vi "Create Map from Values Indexes to Channel and Label Indexes.vi"(8 "error in":errorcluster, 11 "RT hardware channels":T2[](array[typedef]) {"labels settings for RT"."Label Timestamp Channel Data Reference" format="%.0x"; "labels settings for RT"."Word Initial Raw Value" format="%032.0f"; "labels settings for RT"."Label Disable/Trigger Channel Reference" format="%.0x"; "labels settings for RT"."parameter driver data"."Tx parameter refs" format="%.0x"; "labels settings for RT"."parameter driver data"."Rx block data refs"."Data Reference" format="%.0x"; "labels settings for RT"."SDI" format="%02b"; "labels settings for RT"."label" format="%.0o"}) -> (0 "error out":errorcluster, 3 "map":T1)   [LabVIEW 2020, in "Ballard ARINC 429 Engine.lvlib" / "Custom Device.lvlib"]
uses:
  Custom Device.lvlib
  Shared/RT Hardware Channel Settings.ctl
  Shared/RT Label Settings.ctl
  Shared/Label.ctl
  Shared/RT Parameters.ctl
  Shared/Parameter Definition.ctl
  Encoding and Decoding/Encoding.ctl
  <vilib>/NI VeriStand/Custom Device API/Block Data Reference.ctl
  <vilib>/NI VeriStand/Custom Device API/Data Reference.ctl
  <vilib>/NI VeriStand/Custom Device API/Custom Device Item Ref.ctl
  Shared/Transfer Type.ctl
  Shared/Map of Values Indexes to Channel and Label Indexes.ctl
  Encoding and Decoding/Encoding and Decoding.lvlib
  <vilib>/NI VeriStand/Custom Device API/Custom Device API.lvlib
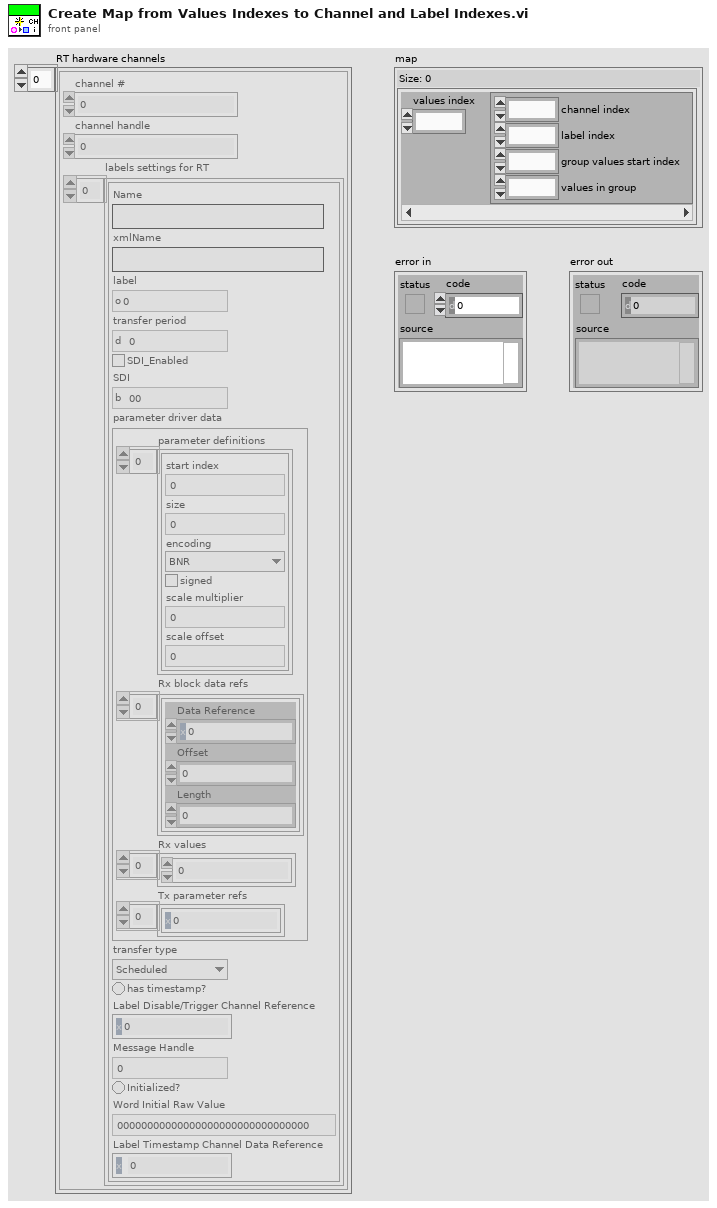
[diagram p1: front panel]
types:
  T1 = typedef "Map of Values Indexes to Channel and Label Indexes.ctl" = map{i32, cluster{"channel index":i32, "label index":i32, "group values start index":i32, "values in group":i32}}
  T2 = typedef "RT Hardware Channel Settings.ctl" = cluster{"channel #":u16, "channel handle":u64, "labels settings for RT":T3[]}
  T3 = typedef "RT Label Settings.ctl" = cluster{"Name":string, "xmlName":string, "label":T4, "transfer period":u32, "SDI_Enabled":bool, "SDI":u8, "parameter driver data":T5, "transfer type":T11, "has timestamp?":bool, "Label Disable/Trigger Channel Reference":T10, "Message Handle":u64, "Initialized?":bool, "Word Initial Raw Value":u32, "Label Timestamp Channel Data Reference":T9}
  T4 = typedef "Label.ctl" = u8
  T5 = typedef "RT Parameters.ctl" = cluster{"parameter definitions":T6[], "Rx block data refs":T8[], "Rx values":dbl[], "Tx parameter refs":T10[]}
  T6 = typedef "Parameter Definition.ctl" = cluster{"start index":i32, "size":i32, "encoding":T7, "signed":bool, "scale multiplier":dbl, "scale offset":dbl}
  T7 = typedef "Encoding and Decoding.lvlib/Encoding.ctl" = enum16{"BNR", "BCD", "Discrete"}
  T8 = typedef "Custom Device API.lvlib/Block Data Reference.ctl" = cluster{"Data Reference":T9, "Offset":u64, "Length":u64}
  T9 = typedef "Custom Device API.lvlib/Data Reference.ctl" = i32
  T10 = typedef "Custom Device API.lvlib/Custom Device Item Ref.ctl" = u64
  T11 = typedef "Transfer Type.ctl" = enum16{"Scheduled", "Acyclic", "Block", "Strobe"}
  T12 = cluster{"channel index":i32, "label index":i32, "group values start index":i32, "values in group":i32}
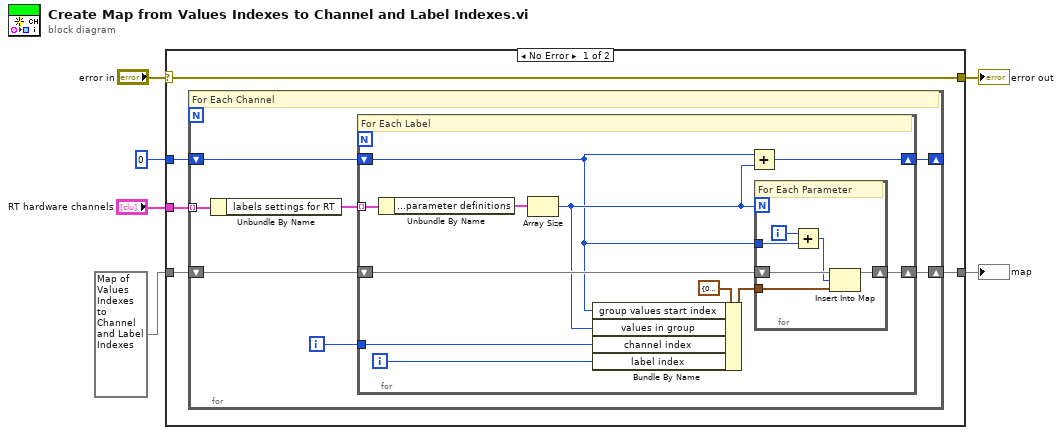
[diagram p0: block diagram]
diagram:
  n1 = case shown="No Error" "error in" {
    selector: "error in" -> [w7 w37]
    tunnel: "RT hardware channels" -> [w11 _]
    tunnel: 0 -> [w10 _]
    tunnel: T1 {} ("map") -> [w9 w36]
    tunnel: [w8 w36] -> w3
    tunnel: [w7 w37] -> w1
    frame No Error {
      n2 = for {
        tunnel: w11 -> [w18] mode=indexing
        shift-right: [w12] -> _
        shift-left: w10 -> [w14]
        shift-right: [w15] -> w8
        shift-left: w9 -> [w16]
        i -> [w13]
        # "For Each Channel"
        n3 = Unbundle By Name(w18) -> ("labels settings for RT"=w17:T3[])
        n4 = for {
          tunnel: w17 -> [w29] mode=indexing
          shift-right: [w26] -> w15
          shift-left: w16 -> [w27]
          tunnel: w13 -> [w25]
          shift-right: [w20] -> w12
          shift-left: w14 -> [w19]
          i -> [w24]
          # "For Each Label"
          n5 = Unbundle By Name(w29) -> ("parameter driver data.parameter definitions"=w28:T6[])
          n6 = Array Size(array=w28) -> (size(s)=w22:i32)
          n7 = Bundle By Name(cluster=T12 {"channel index"=0, "label index"=0, "group values start index"=0, "values in group"=0} ("value"), "group values start index"=w19, "values in group"=w22, "channel index"=w25, "label index"=w24) -> (w21:T12)
          n8 = Add(x=w19, y=w22) -> (x+y=w20:i32)
          n9 = for {
            N: w22 -> [_]
            shift-right: [w34] -> w26
            shift-left: w27 -> [w35]
            tunnel: w19 -> [w32]
            tunnel: w21 -> [w31]
            i -> [w33]
            # "For Each Parameter"
            n10 = Add(x=w33, y=w32) -> (x+y=w30:i32)
            n11 = Insert Into Map(map in=w35, key=w30, value=w31) -> (map out=w34:T1)  [unwired: 2 out]
          }
        }
      }
    }
    frame Error {
    }
  }
  "map" <- w3
  "error out" <- w1
